vi "SVID Declare Notifier.vi"(8 "error in":errorcluster, 11 "SVID Data":T1[](array[typedef])) -> (0 "error out":errorcluster, 3 "SVID Notifier":refnum<notifier>[](array[refnum]))   [LabVIEW 2020, in "SECS Communication.lvlib" / "SECS Data Class.lvclass"]
uses:
  SECS Data Class.lvclass
  SVID Data.ctl
  SECS-II Class/Format Code.ctl
  SECS-II Class/SECS-II Class.lvclass
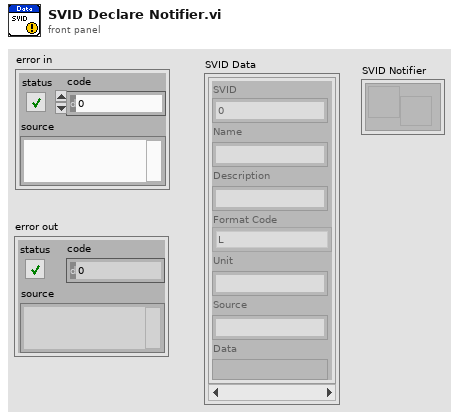
[diagram p1: front panel]
types:
  T1 = typedef "SECS Communication.lvlib/SECS Data Class.lvclass/SVID Data.ctl" = cluster{"SVID":u32, "Name":string, "Description":string, "Format Code":T2, "Unit":string, "Source":string, "Data":variant}
  T2 = typedef "SECS Communication.lvlib/SECS-II Class.lvclass/Format Code.ctl" = enum16{"L", "A", "B", "Boolean", "J", "I1", "I2", "I4", "I8", "U1", "U2", "U4", "U8", "F4", "F8", "Char"}
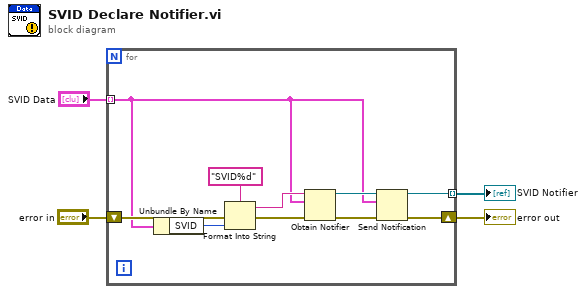
[diagram p0: block diagram]
diagram:
  n1 = for {
    tunnel: "SVID Data" -> [w7] mode=indexing
    shift-right: [w6] -> w2
    shift-left: "error in" -> [w14]
    tunnel: [w5] -> w1 mode=indexing
    n2 = Unbundle By Name(w7) -> ("SVID"=w13:u32)
    n3 = Format Into String(format string="SVID%d", error in=w14, w13) -> (resulting string=w10:string, error out=w11:errorcluster)  [unwired: 1 in]
    n4 = Obtain Notifier(name (unnamed)=w10, notification data type=w7, error in (no error)=w11) -> (notifier out=w9:refnum<notifier>, error out=w8:errorcluster)  [unwired: 1 in, 1 out]
    n5 = Send Notification(notification=w7, notifier=w9, error in (no error)=w8) -> (notifier out=w5:refnum<notifier>, error out=w6:errorcluster)
  }
  "error out" <- w2
  "SVID Notifier" <- w1
